vi "Get Control Offsets by Name and DataType.vi"(6 "offset":i32, 7 "User Specified?":bool, 8 "error in":errorcluster, 9 "Controls":string[](array[string]), 10 "Indicators":string[](array[string]), 11 "bitfile xml in":string) -> (0 "error out":errorcluster, 1 "Control Arrays":T3, 2 "Control Scalars":T1, 3 "Indicator Arrays":T3, 4 "offset past EndTag":i32, 5 "Indicator Scalars":T1)   [LabVIEW 2010, in "FPGA Bitfile Utility.lvlib"]
uses:
  <userlib>/_FPGA Interface Advanced Tools/FPGA Bitfile Utility/FPGA Bitfile Utility.lvlib
  <userlib>/_FPGA Interface Advanced Tools/FPGA Bitfile Utility/TypeDefs/Array Register Set.ctl
  <userlib>/_FPGA Interface Advanced Tools/FPGA Bitfile Utility/TypeDefs/Array Register.ctl
  <userlib>/_FPGA Interface Advanced Tools/FPGA Bitfile Utility/TypeDefs/Scalar Register Set.ctl
  <userlib>/_FPGA Interface Advanced Tools/FPGA Bitfile Utility/TypeDefs/Scalar Register.ctl
  <vilib>/rvi/DataTransferAndStorage/Container/Common/niFpgaDataTypeControl.ctl
  <userlib>/_FPGA Interface Advanced Tools/FPGA Bitfile Utility/Get Register Map.vi
  <userlib>/_FPGA Interface Advanced Tools/FPGA Bitfile Utility/Get Base Address.vi
  <vilib>/rvi/Utilities/XML/nirviXML_GetValue.vi
  <vilib>/rvi/Utilities/XML/nirviXML_GetValue_String.vi
  <vilib>/rvi/Bitfile/niFpgaReadBitfileXml_VIRegisterMap.vi
  <vilib>/rvi/Utilities/XML/nirviXML_GetValue_U32.vi
  <vilib>/Utility/VariantDataType/GetTypeInfo.vi
  <vilib>/Utility/VariantDataType/GetArrayInfo.vi
  <vilib>/Utility/error.llb/Error Cluster From Error Code.vi
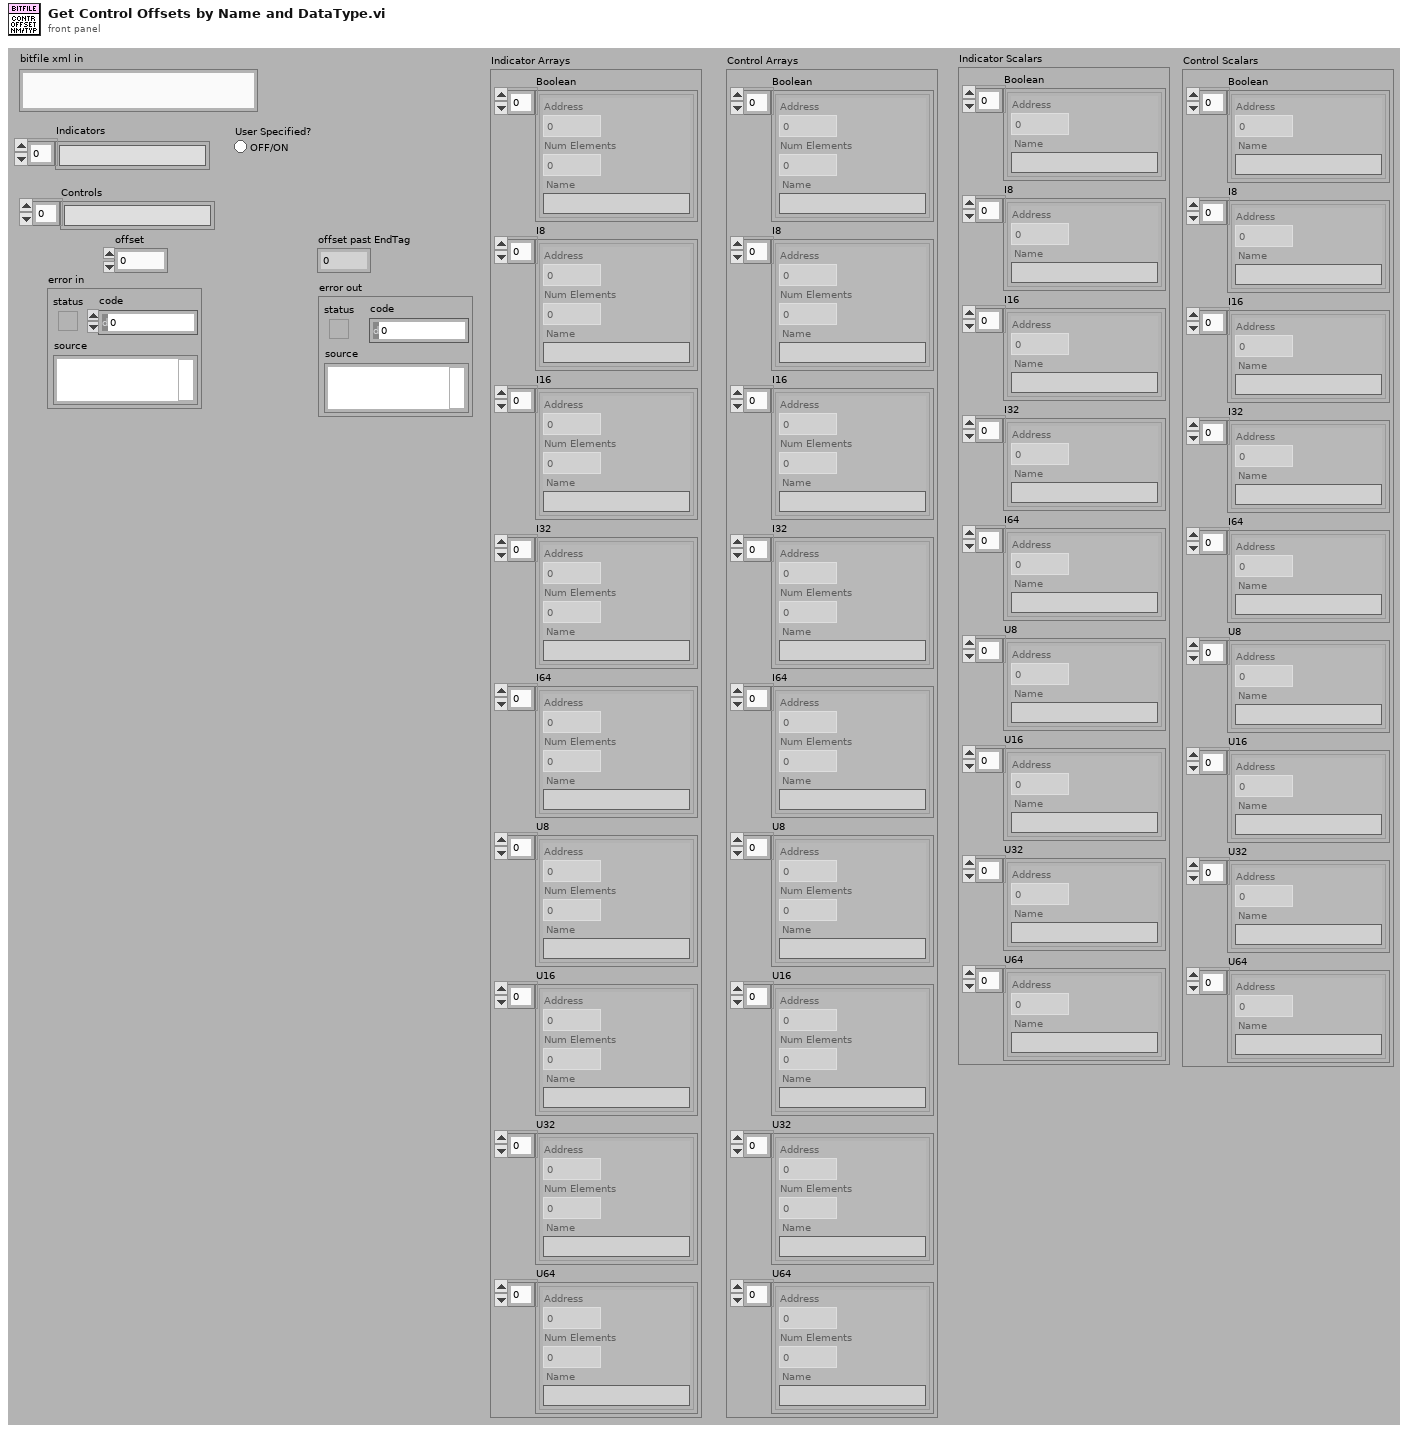
[diagram p1: front panel]
types:
  T1 = typedef "FPGA Bitfile Utility.lvlib/Scalar Register Set.ctl" = cluster{"Boolean":T2[], "I8":T2[], "I16":T2[], "I32":T2[], "I64":T2[], "U8":T2[], "U16":T2[], "U32":T2[], "U64":T2[]}
  T2 = typedef "FPGA Bitfile Utility.lvlib/Scalar Register.ctl" = cluster{"Address":u32, "Name":string}
  T3 = typedef "FPGA Bitfile Utility.lvlib/Array Register Set.ctl" = cluster{"Boolean":T4[], "I8":T4[], "I16":T4[], "I32":T4[], "I64":T4[], "U8":T4[], "U16":T4[], "U32":T4[], "U64":T4[]}
  T4 = typedef "FPGA Bitfile Utility.lvlib/Array Register.ctl" = cluster{"Address":u32, "Num Elements":u32, "Name":string}
  T5 = typedef "FPGA Bitfile Utility.lvlib/Control_Indicator Info.ctl" = cluster{"Array?":bool, "Data Type":T6, "Address":u32, "Num Elements":u32, "Name":string}
  T6 = typedef "niFpgaDataTypeControl.ctl" = enum32{"Boolean", "I8", "I16", "I32", "I64", "U8", "U16", "U32", "U64", "FXP", "CustomControl"}
  T7 = cluster{"Address":u32, "Num Elements":u32, "Name":string}
  T8 = cluster{T4[], T4[], T4[], T4[], T4[], T4[], T4[], T4[], T4[]}
  T9 = cluster{T2[], T2[], T2[], T2[], T2[], T2[], T2[], T2[], T2[]}
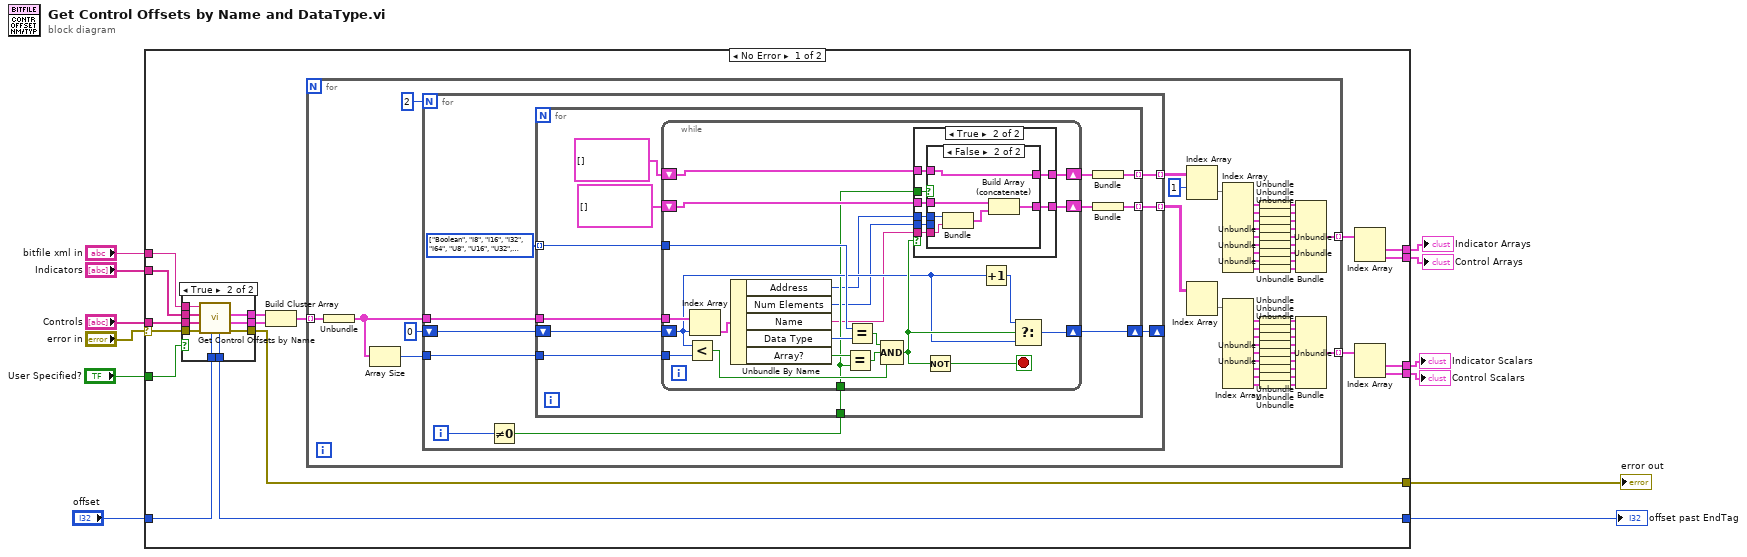
[diagram p0: block diagram]
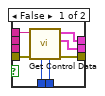
[diagram p2: hidden frame]
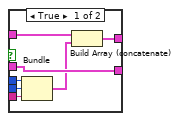
[diagram p4: hidden frame]
diagram:
  n1 = case shown="No Error" "error in" {
    selector: "error in" -> [w25 w161]
    tunnel: [w28 _] -> w2
    tunnel: [w27 _] -> w3
    tunnel: [w26 _] -> w4
    tunnel: [w21 w161] -> w11
    tunnel: "bitfile xml in" -> [w24 _]
    tunnel: [w20 w160] -> w9
    tunnel: "offset" -> [w19 w160]
    tunnel: "Controls" -> [w18 _]
    tunnel: "Indicators" -> [w17 _]
    tunnel: [w14 _] -> w5
    tunnel: "User Specified?" -> [w13 _]
    frame No Error {
      n2 = case shown="True" w13 {
        tunnel: w25 -> [w35 w45]
        tunnel: w24 -> [w36 w44]
        tunnel: [w31 w43] -> w23
        tunnel: [w30 w42] -> w22
        tunnel: [w32 w41] -> w21
        tunnel: [w33 w40] -> w20
        tunnel: w19 -> [w34 w39]
        tunnel: w18 -> [_ w38]
        tunnel: w17 -> [_ w37]
        frame False {
          n3 = call <userlib>:"Get Control Data.vi"("offset"=w34, "error in (no error)"=w35, "bitfile xml in"=w36) -> ("error out"=w32:errorcluster, "Controls"=w30:T5[], "Indicators"=w31:T5[], "offset past EndTag"=w33:i32)  [unwired: 5 in]
        }
        frame True {
          n4 = call <userlib>:"Get Control Offsets by Name.vi"("offset"=w39, "error in (no error)"=w45, "Controls"=w38, "Indicators"=w37, "bitfile xml in"=w44) -> ("error out"=w41:errorcluster, "Control Offsets"=w42:T5[], "Indicator Offsets"=w43:T5[], "offset past EndTag"=w40:i32)  [unwired: 3 in]
        }
      }
      n5 = Build Cluster Array(w23, w22) -> (w29:cluster{"Control Offsets":T5[]}[])
      n6 = for {
        tunnel: w29 -> [w93] mode=indexing
        tunnel: [w48] -> w15 mode=indexing
        tunnel: [w47] -> w16 mode=indexing
        n7 = Unbundle(w93) -> ("Control Offsets"=w91:T5[])
        n8 = Array Size(array=w91) -> (size(s)=w90:i32)
        n9 = for {
          N: 2 -> [_]
          tunnel: w91 -> [w102]
          shift-right: [w99] -> _
          shift-left: 0 -> [w100]
          tunnel: w90 -> [w96]
          tunnel: [w95] -> w87 mode=indexing
          tunnel: [w94] -> w88 mode=indexing
          i -> [w101]
          w97 = T6[] [enum."Boolean", enum."I8", enum."I16", enum."I32", enum."I64", enum."U8", enum."U16", enum."U32", enum."U64"] items=["Boolean", "I8", "I16", "I32", "I64", "U8", "U16", "U32", "U64", "FXP", "CustomControl"]
          n10 = Not Equal To 0?(x=w101) -> (x != 0?=w98:bool)
          n11 = for {
            tunnel: w97 -> [w114] mode=indexing
            tunnel: w102 -> [w113]
            tunnel: w98 -> [w110]
            shift-right: [w111] -> w99
            shift-left: w100 -> [w112]
            tunnel: [w107] -> w95 mode=indexing
            tunnel: w96 -> [w106]
            tunnel: [w103] -> w94 mode=indexing
            n12 = while {
              tunnel: w114 -> [w131]
              tunnel: w113 -> [w136]
              shift-right: [w134] -> w111
              shift-left: w112 -> [w122]
              tunnel: w110 -> [w120]
              shift-right: [w128] -> w109
              shift-left: T2[] [] -> [w127]
              tunnel: w106 -> [w124]
              shift-right: [w116] -> w104
              shift-left: T4[] [] -> [w115]
              stop <- w125 stop-if-true
              n13 = Less?(x=w122, y=w124) -> (x < y?=w123:bool)
              n14 = Index Array(array=w136, index=w122) -> (element=w129:T5)
              n15 = Unbundle By Name(w129) -> ("Address"=w118:u32, "Num Elements"=w117:u32, "Name"=w119:string, "Data Type"=w132:T6, "Array?"=w133:bool)
              n16 = Equal?(x=w133, y=w120) -> (x = y?=w121:bool)
              n17 = Equal?(x=w131, y=w132) -> (x = y?=w130:bool)
              n18 = Compound Arithmetic op=AND(w130, w121, w123) -> (w126:bool)
              n19 = case shown="True" w126 {
                tunnel: [w138 w146] -> w128
                tunnel: w127 -> [w138 w145]
                tunnel: w120 -> [_ w144]
                tunnel: w118 -> [_ w143]
                tunnel: w119 -> [_ w142]
                tunnel: w117 -> [_ w141]
                tunnel: [w137 w140] -> w116
                tunnel: w115 -> [w137 w139]
                frame False {
                }
                frame True {
                  n20 = case shown="False" w144 {
                    tunnel: [w150 w159] -> w146
                    tunnel: w145 -> [w150 w158]
                    tunnel: w143 -> [w153 w157]
                    tunnel: w142 -> [w152 w156]
                    tunnel: w141 -> [w151 _]
                    tunnel: [w149 w154] -> w140
                    tunnel: w139 -> [w148 w154]
                    frame True {
                      n21 = Bundle("Address"=w153, "Num Elements"=w151, "Name"=w152) -> (w147:T7)  [unwired: 1 in]
                      n22 = Build Array (concatenate)(w148, w147) -> (w149:T4[])
                    }
                    frame False {
                      n23 = Bundle("Address"=w157, "Name"=w156) -> (w155:cluster{"Address":u32, "Name":string})  [unwired: 1 in]
                      n24 = Build Array (concatenate)(w158, w155) -> (w159:T2[])
                    }
                  }
                }
              }
              n25 = Not(x=w126) -> (.not. x?=w125:bool)
              n26 = Increment(x=w122) -> (x+1=w135:i32)
              n27 = Select(t=w135, s=w126, f=w122) -> (s? t:f=w134:i32)
            }
            n28 = Bundle(w104) -> (w103:cluster{T4[]})  [unwired: 1 in]
            n29 = Bundle(w109) -> (w107:cluster{T2[]})  [unwired: 1 in]
          }
        }
        n30 = Index Array(array=w88, index (row)=1) -> (element=w68:cluster{T4[]}[])  [unwired: 1 in]
        n31 = Index Array(array=w87) -> (element=w49:cluster{T2[]}[])  [unwired: 2 in]
        n32 = Index Array(array=w68) -> (element #1=w69:cluster{T4[]}, element #2=w71:cluster{T4[]}, element #3=w73:cluster{T4[]}, element #4=w74:cluster{T4[]}, element #5=w77:cluster{T4[]}, element #6=w78:cluster{T4[]}, element #7=w79:cluster{T4[]}, element #8=w80:cluster{T4[]}, element #9=w81:cluster{T4[]})  [unwired: 9 in]
        n33 = Index Array(array=w49) -> (element #1=w67:cluster{T2[]}, element #2=w65:cluster{T2[]}, element #3=w63:cluster{T2[]}, element #4=w62:cluster{T2[]}, element #5=w59:cluster{T2[]}, element #6=w58:cluster{T2[]}, element #7=w57:cluster{T2[]}, element #8=w56:cluster{T2[]}, element #9=w55:cluster{T2[]})  [unwired: 9 in]
        n34 = Unbundle(w69) -> (w70:T4[])
        n35 = Unbundle(w71) -> (w72:T4[])
        n36 = Unbundle(w73) -> (w76:T4[])
        n37 = Unbundle(w74) -> (w75:T4[])
        n38 = Unbundle(w77) -> (w86:T4[])
        n39 = Unbundle(w78) -> (w85:T4[])
        n40 = Unbundle(w79) -> (w84:T4[])
        n41 = Unbundle(w80) -> (w83:T4[])
        n42 = Unbundle(w81) -> (w82:T4[])
        n43 = Unbundle(w67) -> (w66:T2[])
        n44 = Unbundle(w65) -> (w64:T2[])
        n45 = Unbundle(w63) -> (w60:T2[])
        n46 = Unbundle(w62) -> (w61:T2[])
        n47 = Unbundle(w59) -> (w50:T2[])
        n48 = Unbundle(w58) -> (w51:T2[])
        n49 = Unbundle(w57) -> (w52:T2[])
        n50 = Unbundle(w56) -> (w53:T2[])
        n51 = Unbundle(w55) -> (w54:T2[])
        n52 = Bundle(w70, w72, w76, w75, w86, w85, w84, w83, w82) -> (w47:T8)  [unwired: 1 in]
        n53 = Bundle(w66, w64, w60, w61, w50, w51, w52, w53, w54) -> (w48:T9)  [unwired: 1 in]
      }
      n54 = Index Array(array=w16) -> (element #1=w14:T8, element #2=w26:T8)  [unwired: 2 in]
      n55 = Index Array(array=w15) -> (element #1=w27:T9, element #2=w28:T9)  [unwired: 2 in]
    }
    frame Error {
    }
  }
  "error out" <- w11
  "offset past EndTag" <- w9
  "Indicator Arrays" <- w5
  "Control Arrays" <- w4
  "Indicator Scalars" <- w3
  "Control Scalars" <- w2
